vi "RGBaHVS.vi"() -> ()   [LabVIEW 2020]
panel:
  out "Color":u32(colorbox)
  out "H":dbl(knob) scale format="%#_5g"
  out "V":dbl(slide) scale=0.0..1.0
  out "S":dbl(slide) scale=0.0..1.0
  in  "B":u8(slide) scale=0.0..255.0
  in  "G":u8(slide) scale=0.0..255.0
  in  "R":u8(slide) scale=0.0..255.0
  # "Ceballos Conde Emanuel"
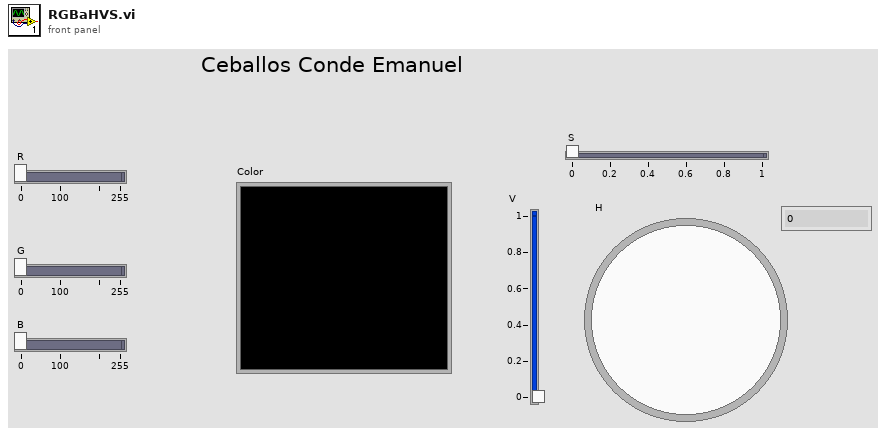
[diagram p1: front panel]
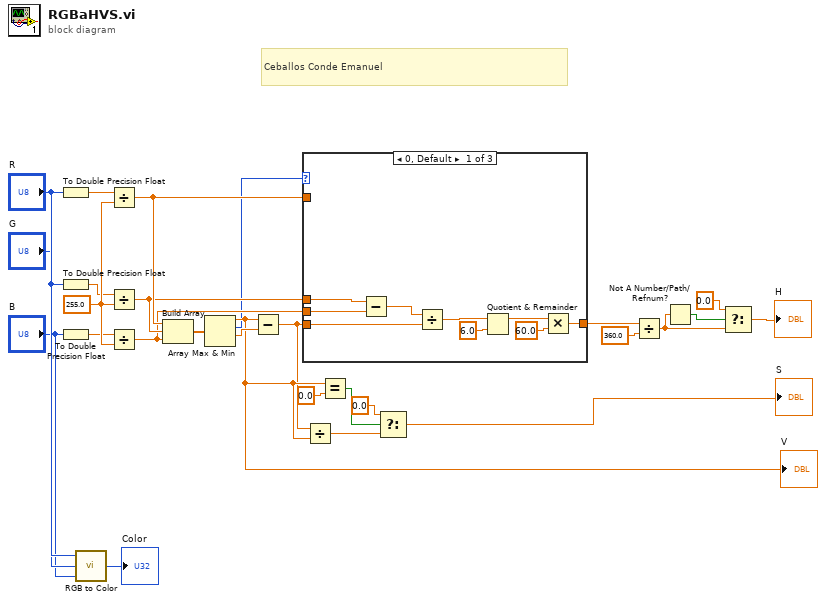
[diagram p0: block diagram]
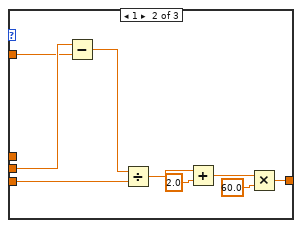
[diagram p2: hidden frame]
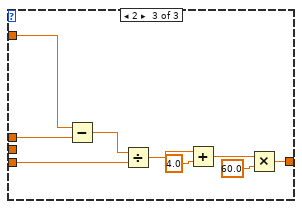
[diagram p3: hidden frame]
diagram:
  w27 = 255.0 ("y")
  # "Ceballos Conde Emanuel"
  n1 = To Double Precision Float(number="R") -> (double precision float=w26:dbl)
  n2 = To Double Precision Float(number="G") -> (double precision float=w25:dbl)
  n3 = To Double Precision Float(number="B") -> (double precision float=w24:dbl)
  n4 = call <vilib>:"RGB to Color.vi"("B"="B", "G"="G", "R"="R") -> ("Color"=→"Color":u32)
  n5 = Divide(x=w26, y=w27) -> (x/y=w8:dbl)
  n6 = Divide(x=w25, y=w27) -> (x/y=w7:dbl)
  n7 = Divide(x=w24, y=w27) -> (x/y=w6:dbl)
  n8 = Build Array(w8, w7, w6) -> (w23:dbl[])
  n9 = Array Max & Min(array=w23) -> (max value=w13:dbl, max index (indices)=w1:i32, min value=w19:dbl)  [unwired: 1 out]
  "V" <- w13
  n10 = Subtract(x=w13, y=w19) -> (x-y=w11:dbl)
  n11 = case shown="0, Default" w1 {
    tunnel: [w30 w39 w48] -> w10
    tunnel: w7 -> [w29 _ w46]
    tunnel: w6 -> [w28 w38 _]
    tunnel: w11 -> [w35 w44 w53]
    tunnel: w8 -> [_ w37 w47]
    frame 0, Default {
      n12 = Subtract(x=w29, y=w28) -> (x-y=w36:dbl)
      n13 = Divide(x=w36, y=w35) -> (x/y=w34:dbl)
      n14 = Quotient & Remainder(x=w34, y=6.0) -> (x-y*floor(x/y)=w31:dbl)  [unwired: 1 out]
      n15 = Multiply(x=w31, y=60.0) -> (x*y=w30:dbl)
    }
    frame 1 {
      n16 = Subtract(x=w38, y=w37) -> (x-y=w45:dbl)
      n17 = Divide(x=w45, y=w44) -> (x/y=w43:dbl)
      n18 = Add(x=w43, y=2.0) -> (x+y=w40:dbl)
      n19 = Multiply(x=w40, y=60.0) -> (x*y=w39:dbl)
    }
    frame 2 {
      n20 = Subtract(x=w47, y=w46) -> (x-y=w54:dbl)
      n21 = Divide(x=w54, y=w53) -> (x/y=w52:dbl)
      n22 = Add(x=w52, y=4.0) -> (x+y=w49:dbl)
      n23 = Multiply(x=w49, y=60.0) -> (x*y=w48:dbl)
    }
  }
  n24 = Divide(x=w11, y=w13) -> (x/y=w18:dbl)
  n25 = Equal?(x=w13, y=0.0) -> (x = y?=w21:bool)
  n26 = Select(t=0.0, s=w21, f=w18) -> (s? t:f=→"S":dbl)
  n27 = Divide(x=w10, y=360.0) -> (x/y=w4:dbl)
  n28 = Not A Number/Path/Refnum?(number/path/refnum=w4) -> (NaN/Path/Refnum?=w5:bool)
  n29 = Select(t=0.0, s=w5, f=w4) -> (s? t:f=→"H":dbl)
